vi "rosbridge_write.vi"(8 "error in (no error)":errorcluster, 9 "JSON string":string, 10 "stop":bool, 11 "TCP Network Connection in":refnum<k5>) -> (0 "error out":errorcluster, 3 "TCP Network Connection out":refnum<k5>)   [LabVIEW 2013]
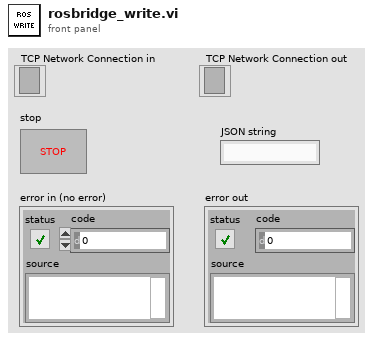
[diagram p1: front panel]
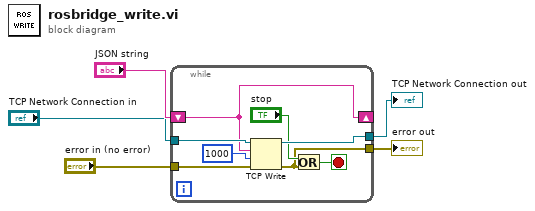
[diagram p0: block diagram]
diagram:
  n1 = while {
    tunnel: [w12] -> w2
    tunnel: "TCP Network Connection in" -> [w9]
    tunnel: "error in (no error)" -> [w10]
    shift-right: [w6] -> _
    shift-left: "JSON string" -> [w6]
    tunnel: [w7] -> w1
    stop <- w13 stop-if-true
    n2 = TCP Write(connection ID=w9, data in=w6, error in (no error)=w10, 9:1000 ("timeout ms (25000)")) -> (connection ID out=w12:refnum<k5>, error out=w7:errorcluster)  [unwired: 1 out]
    n3 = Or(x="stop", y=w7) -> (x .or. y?=w13:bool)
  }
  "error out" <- w1
  "TCP Network Connection out" <- w2
